vi "SeqMgr.Variables - Init.vi"(8 "error in (no error)":errorcluster, 10 "Vars":variant, 11 "SeqMgr in":refnum<class "SeqMgr.lvclass">) -> (0 "error out":errorcluster, 3 "SeqMgr out":refnum<class "SeqMgr.lvclass">)   [LabVIEW 2024, in "EQMF.lvlib" / "SeqMgr.lvlib" / "SeqMgr.lvclass"]
uses:
  SeqMgr.lvclass
  SeqMgr.lvclass/SeqMgr.ctl
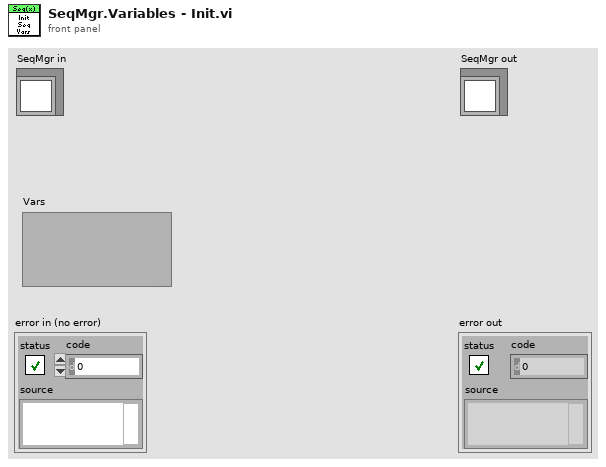
[diagram p1: front panel]
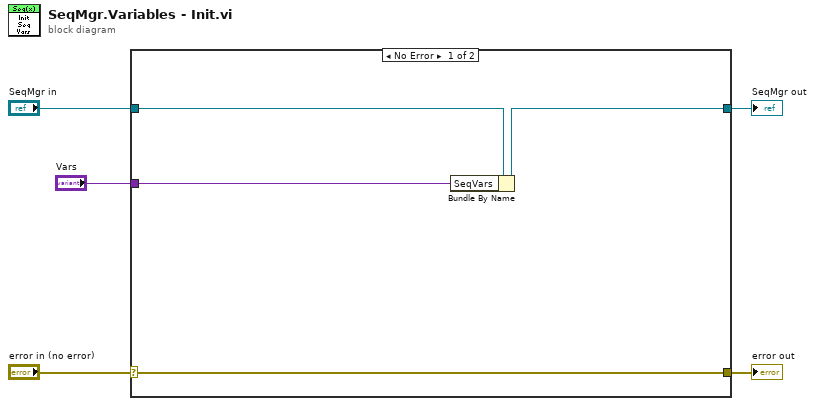
[diagram p0: block diagram]
diagram:
  n1 = case shown="No Error" "error in (no error)" {
    selector: "error in (no error)" -> [w9 w11]
    tunnel: [w9 w11] -> w4
    tunnel: [w7 w10] -> w2
    tunnel: "SeqMgr in" -> [w8 w10]
    tunnel: "Vars" -> [w6 _]
    frame No Error {
      n2 = Bundle By Name(cluster=w8, "SeqVars"=w6) -> (w7:refnum<class "SeqMgr.lvclass">)
    }
    frame Error {
    }
  }
  "error out" <- w4
  "SeqMgr out" <- w2
